vi "SP Format Fundamental Value for Display (complex array).vi"(4 "dF, MHz":dbl, 8 "Sxx Measured Format":T1, 9 "Fundamental Values":cdb[](array[numeric])) -> (1 "Formatted Values":dbl[](array[numeric]))   [LabVIEW 2011]
uses:
  TypeDefs/SP Format.ctl
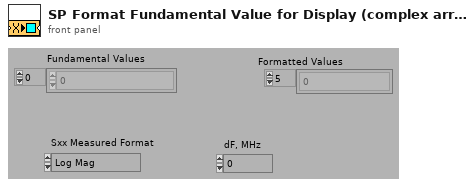
[diagram p1: front panel]
types:
  T1 = typedef "SP Format.ctl" = enum16{"Log Mag", "Lin Mag", "SWR", "Phase", "Expanded Phase", "Delay", "Insertion Loss", "Isolation", "Return Loss"}
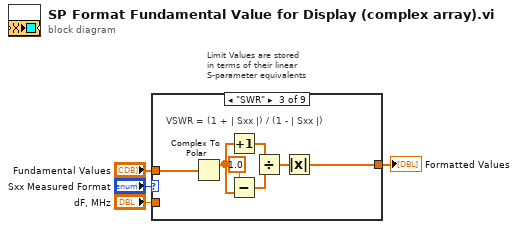
[diagram p0: block diagram]
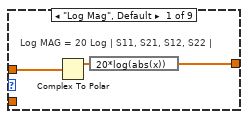
[diagram p2: hidden frame]
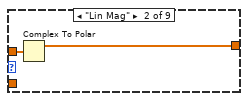
[diagram p3: hidden frame]
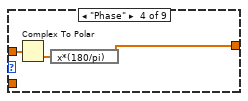
[diagram p4: hidden frame]
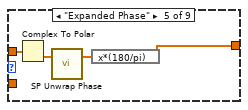
[diagram p5: hidden frame]
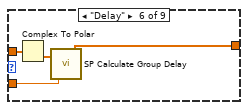
[diagram p6: hidden frame]
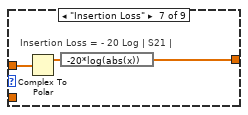
[diagram p7: hidden frame]
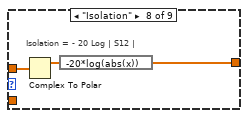
[diagram p8: hidden frame]
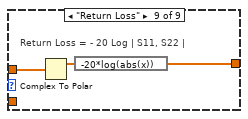
[diagram p9: hidden frame]
diagram:
  # "Limit Values are stored\nin terms of their linear\nS-parameter equivalents"
  n1 = case shown="\"SWR\"" "Sxx Measured Format" {
    tunnel: [w5 w8 w10 w17 w22 w24 w28 w31 w34] -> w2
    tunnel: "Fundamental Values" -> [w7 w9 w12 w19 w23 w27 w30 w32 w35]
    tunnel: "dF, MHz" -> [_ _ _ _ _ w25 _ _ _]
    frame "Log Mag", Default {
      # "Log MAG = 20 Log | S11, S21, S12, S22 |"
      n2 = Complex To Polar(r * e^(i*theta)=w7) -> (r=w6:dbl[])  [unwired: 1 out]
      n3 = expression code="20*log(abs(x))"(w6) -> (w5:dbl[])
    }
    frame "Lin Mag" {
      n4 = Complex To Polar(r * e^(i*theta)=w9) -> (r=w8:dbl[])  [unwired: 1 out]
    }
    frame "SWR" {
      # "VSWR = (1 + | Sxx |) / (1 - | Sxx |)"
      n5 = Complex To Polar(r * e^(i*theta)=w12) -> (r=w11:dbl[])  [unwired: 1 out]
      n6 = Increment(x=w11) -> (x+1=w16:dbl[])
      n7 = Subtract(x=1.0, y=w11) -> (x-y=w14:dbl[])
      n8 = Divide(x=w16, y=w14) -> (x/y=w13:dbl[])
      n9 = Absolute Value(x=w13) -> (abs(x)=w10:dbl[])
    }
    frame "Phase" {
      n10 = Complex To Polar(r * e^(i*theta)=w19) -> (theta=w18:dbl[])  [unwired: 1 out]
      n11 = expression code="x*(180/pi)"(w18) -> (w17:dbl[])
    }
    frame "Expanded Phase" {
      n12 = Complex To Polar(r * e^(i*theta)=w23) -> (theta=w20:dbl[])  [unwired: 1 out]
      n13 = call "SP Unwrap Phase.vi"("Phase"=w20) -> ("Unwrapped Phase"=w21:dbl[])  [unwired: 1 out]
      n14 = expression code="x*(180/pi)"(w21) -> (w22:dbl[])
    }
    frame "Delay" {
      n15 = Complex To Polar(r * e^(i*theta)=w27) -> (theta=w26:dbl[])  [unwired: 1 out]
      n16 = call "SP Calculate Group Delay.vi"("dF, MHz"=w25, "Phase, radians"=w26) -> ("Group Delay, seconds"=w24:dbl[])  [unwired: 1 out]
    }
    frame "Insertion Loss" {
      # "Insertion Loss = - 20 Log | S21 |"
      n17 = Complex To Polar(r * e^(i*theta)=w30) -> (r=w29:dbl[])  [unwired: 1 out]
      n18 = expression code="-20*log(abs(x))"(w29) -> (w28:dbl[])
    }
    frame "Isolation" {
      # "Isolation = - 20 Log | S12 |"
      n19 = Complex To Polar(r * e^(i*theta)=w32) -> (r=w33:dbl[])  [unwired: 1 out]
      n20 = expression code="-20*log(abs(x))"(w33) -> (w31:dbl[])
    }
    frame "Return Loss" {
      # "Return Loss = - 20 Log | S11, S22 |"
      n21 = Complex To Polar(r * e^(i*theta)=w35) -> (r=w36:dbl[])  [unwired: 1 out]
      n22 = expression code="-20*log(abs(x))"(w36) -> (w34:dbl[])
    }
  }
  "Formatted Values" <- w2
